vi "createNotifierStopServer.vi"(8 "error in (no error)":errorcluster, 11 "tcpServerBase in":refnum<class "TcpServerBase.lvclass">) -> (0 "error out":errorcluster, 3 "tcpServerBase out":refnum<class "TcpServerBase.lvclass">)   [LabVIEW 2018, in "TcpServerBase.lvclass"]
doc: "Create the notifierStopServer reference to stop the TcpServer."
uses:
  TcpServerBase.lvclass
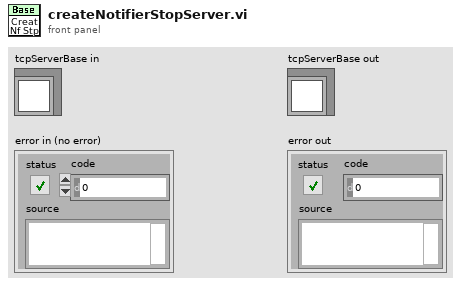
[diagram p1: front panel]
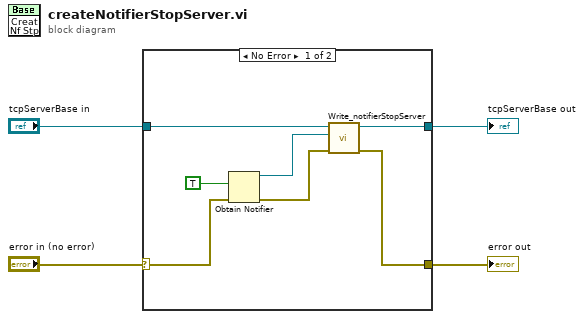
[diagram p0: block diagram]
diagram:
  n1 = case shown="No Error" "error in (no error)" {
    selector: "error in (no error)" -> [w11 w13]
    tunnel: "tcpServerBase in" -> [w10 w12]
    tunnel: [w8 w12] -> w3
    tunnel: [w7 w13] -> w1
    frame No Error {
      n2 = Obtain Notifier(notification data type=TRUE, error in (no error)=w11) -> (notifier out=w5:refnum<notifier>, error out=w9:errorcluster)  [unwired: 2 in, 1 out]
      n3 = call "Write_notifierStopServer.vi"("error in (no error)"=w9, "notifierStopServer"=w5, "TcpServerBase in"=w10) -> ("error out"=w7:errorcluster, "TcpServerBase out"=w8:refnum<class "TcpServerBase.lvclass">)  [unwired: 7 in]
    }
    frame Error {
    }
  }
  "error out" <- w1
  "tcpServerBase out" <- w3
